vi "Diagram Connect Tunnel with Wire.vi"(8 "error in (no error)":errorcluster, 9 "FrontEnd Connected Info":T1[](array[typedef]), 10 "Front Tunnels":refnum<vi>[](array[refnum]), 11 "Diagram in":refnum<vi>) -> (0 "error out":errorcluster, 2 "Array out":i32[](array[numeric]), 3 "Diagram out":refnum<vi>)   [LabVIEW 2017, in "CSM-Helper.lvclass"]
uses:
  CSM-Helper.lvclass
  Typedef/Def-Conncted Information.ctl
  <vilib>/Utility/miscctls.llb/LVPositionTypeDef.ctl
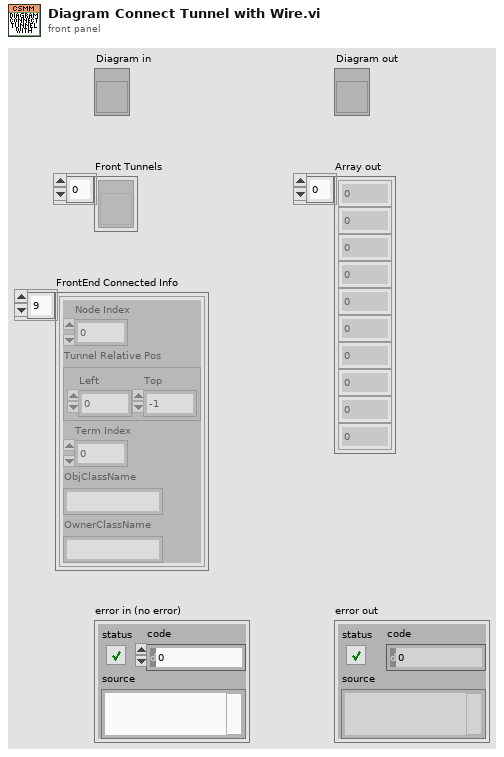
[diagram p1: front panel]
types:
  T1 = typedef "CSM-Helper.lvclass/Def-Conncted Information.ctl" = cluster{"Node Index":i32, "Tunnel Relative Pos":T2, "Term Index":i32, "ObjClassName":string, "OwnerClassName":string}
  T2 = typedef "LVPositionTypeDef.ctl" = cluster{"Left":i32, "Top":i32}
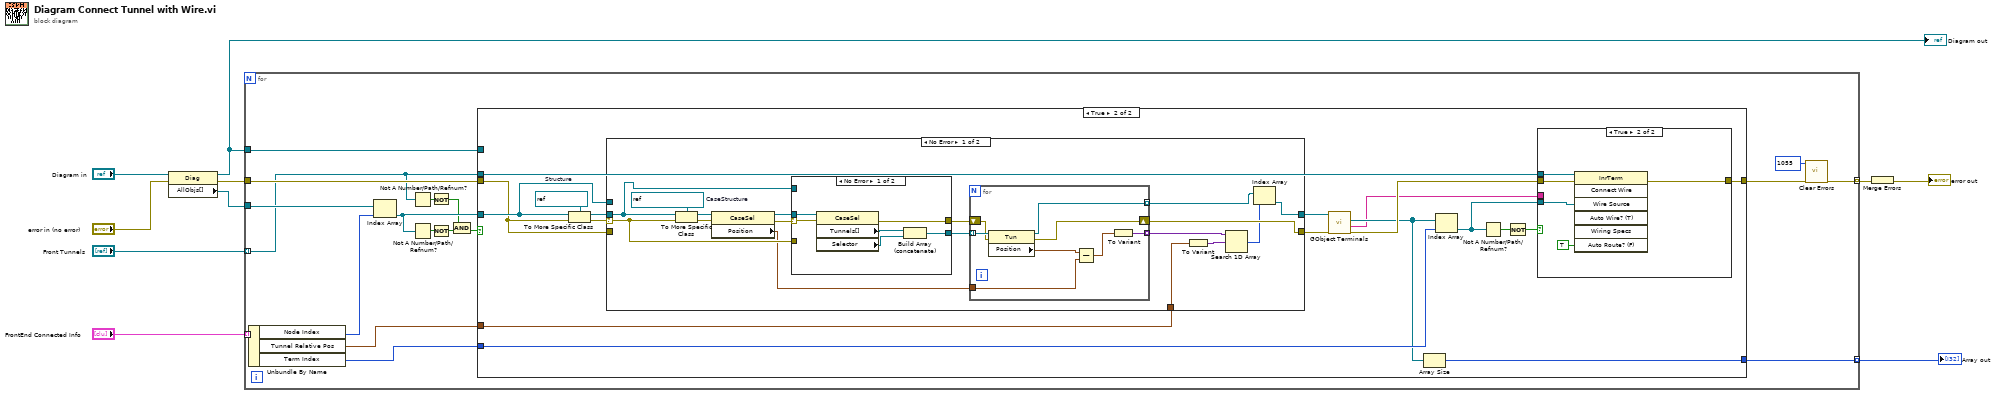
[diagram p0: block diagram]
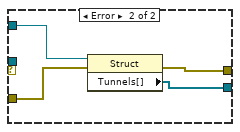
[diagram p3: hidden frame]
diagram:
  n1 = property on="Property Node" class="Diag"(reference="Diagram in", error in="error in (no error)") -> (reference out=w8:refnum<vi>, error out=w10:errorcluster, "AllObjs[]"=w1:refnum<vi>[])
  "Diagram out" <- w8
  n2 = for {
    tunnel: w1 -> [w26]
    tunnel: "FrontEnd Connected Info" -> [w25] mode=indexing
    tunnel: "Front Tunnels" -> [w13] mode=indexing
    tunnel: w10 -> [w28]
    tunnel: [w16] -> w2 mode=indexing
    tunnel: [w22] -> w6 mode=indexing
    tunnel: w8 -> [w21]
    n3 = Unbundle By Name(w25) -> ("Node Index"=w19:i32, "Tunnel Relative Pos"=w17:T2, "Term Index"=w18:i32)
    n4 = Index Array(array=w26, index=w19) -> (element=w23:refnum<vi>)
    n5 = Not A Number/Path/Refnum?(number/path/refnum=w13) -> (NaN/Path/Refnum?=w14:bool)
    n6 = Not A Number/Path/Refnum?(number/path/refnum=w23) -> (NaN/Path/Refnum?=w20:bool)
    n7 = Not(x=w14) -> (.not. x?=w11:bool)
    n8 = Not(x=w20) -> (.not. x?=w24:bool)
    n9 = And(x=w11, y=w24) -> (x .and. y?=w12:bool)
    n10 = case shown="True" w12 {
      tunnel: w28 -> [w29 w31]
      tunnel: [w29 w47] -> w27
      tunnel: w23 -> [_ w32]
      tunnel: w13 -> [_ w45]
      tunnel: [_ w46] -> w22
      tunnel: w21 -> [_ _]
      tunnel: w18 -> [_ w44]
      tunnel: w17 -> [_ w34]
      frame False {
      }
      frame True {
        w37 = refnum<vi> refnum  # Structure
        n11 = To More Specific Class(target class=w37, reference=w32, error in=w31) -> (specific class reference=w38:refnum<vi>, error out=w35:errorcluster)
        n12 = case shown="No Error" w35 {
          selector: w35 -> [w61 _]
          tunnel: w38 -> [w62 _]
          tunnel: [w48 w84] -> w36
          tunnel: w34 -> [w53 _]
          tunnel: [w58 w83] -> w33
          tunnel: w32 -> [_ w84]
          tunnel: w31 -> [_ w83]
          frame No Error {
            w63 = refnum<vi> refnum  # CaseStructure
            n13 = To More Specific Class(target class=w63, reference=w62, error in=w61) -> (specific class reference=w64:refnum<vi>, error out=w56:errorcluster)
            n14 = property class="CaseSel"(reference=w64, error in=w56) -> (reference out=w57:refnum<vi>, error out=w55:errorcluster, "Position"=w54:T2)
            n15 = case shown="No Error" w55 {
              selector: w55 -> [w76 _]
              tunnel: [w77 w82] -> w59
              tunnel: w57 -> [w75 _]
              tunnel: [w74 w79] -> w60
              tunnel: w62 -> [_ w81]
              tunnel: w61 -> [_ w80]
              frame No Error {
                n16 = property class="CaseSel"(reference=w75, error in=w76) -> (error out=w77:errorcluster, "Tunnels[]"=w78:refnum<vi>[], "Selector"=w73:refnum<vi>)  [unwired: 1 out]
                n17 = Build Array (concatenate)(w78, w73) -> (w74:refnum<vi>[])
              }
              frame Error {
                n18 = property class="Struct"(reference=w81, error in=w80) -> (error out=w82:errorcluster, "Tunnels[]"=w79:refnum<vi>[])  [unwired: 1 out]
              }
            }
            n19 = for {
              tunnel: w60 -> [w72] mode=indexing
              tunnel: [w66] -> w52 mode=indexing
              shift-right: [w70] -> w58
              shift-left: w59 -> [w71]
              tunnel: w54 -> [w68]
              tunnel: [w65] -> w50 mode=indexing
              n20 = property class="Tun"(reference=w72, error in=w71) -> (reference out=w65:refnum<vi>, error out=w70:errorcluster, "Position"=w69:T2)
              n21 = Subtract(x=w69, y=w68) -> (x-y=w67:T2)
              n22 = To Variant(anything=w67) -> (Variant=w66:variant)
            }
            n23 = To Variant(anything=w53) -> (Variant=w51:variant)
            n24 = Search 1D Array(1D array=w52, element=w51) -> (index of element=w49:i32)  [unwired: 1 in]
            n25 = Index Array(array=w50, index=w49) -> (element=w48:refnum<vi>)
          }
          frame Error {
          }
        }
        n26 = call "GObject Terminals.vi"("error in (no error)"=w33, "GObject in"=w36) -> ("error in (no error) (dup)"=w40:errorcluster, "Class Name"=w30:string, "Terms[]"=w39:refnum<vi>[])  [unwired: 5 in, 2 out]
        n27 = Array Size(array=w39) -> (size(s)=w46:i32)
        n28 = Index Array(array=w39, index=w44) -> (element=w41:refnum<vi>)
        n29 = Not A Number/Path/Refnum?(number/path/refnum=w41) -> (NaN/Path/Refnum?=w43:bool)
        n30 = Not(x=w43) -> (.not. x?=w42:bool)
        n31 = case shown="True" w42 {
          tunnel: w40 -> [w85 w90]
          tunnel: [w85 w86] -> w47
          tunnel: w45 -> [_ w88]
          tunnel: w41 -> [_ w87]
          tunnel: w30 -> [_ _]
          frame False {
          }
          frame True {
            n32 = invoke class="InrTerm" method="Connect Wire"(reference=w88, error in=w90, "Wire Source"=w87, "Auto Route? (F)"=TRUE) -> (error out=w86:errorcluster)  [unwired: 3 in, 6 out]
          }
        }
      }
    }
    n33 = call <vilib>:"Clear Errors.vi"("error in (no error)"=w27, "specific error code to clear (0: all)"=1055) -> ("error out"=w16:errorcluster)  [unwired: 4 in, 1 out]
  }
  "Array out" <- w6
  n34 = Merge Errors(w2) -> (→"error out":errorcluster)
